vi "DefaultFromINI.vi"(8 "error in (no error)":errorcluster, 11 "ChromaPowerSupply":refnum<class "ChromaPowerSupply.lvclass">) -> (0 "error out":errorcluster, 3 "ChromaPowerSupply":refnum<class "ChromaPowerSupply.lvclass">)   [LabVIEW 2018, in "AcPwrPlugins.lvlib" / "ChromaPowerSupply.lvclass"]
doc: "This VI loads the instruments' configuration previously stored on file."
uses:
  ChromaPowerSupply.lvclass
  C:/Program Files (x86)/National Instruments/LabVIEW 2018/user.lib/NIST/BaseClasses/BasePlugin_class/BasePlugin.lvclass
  C:/Users/Public/Projects/ICDAS/NistPluggableModules/AcPwr/AcPwrPlugins/AcPwrBaseClass/AcPwrBase.lvclass
  TypeDefs/Device(s)Settings.ctl
  TypeDefs/Measurements.ctl
  <userlib>/NIST/BaseClasses/BasePlugin_class/BasePlugin.lvclass/BasePlugin.ctl
  <userlib>/NIST/BaseClasses/BasePlugin_class/Accessors/Read PluginIniFilePath.vi
  AcPwrBaseClass/AcPwrBase.lvclass
  <vilib>/Utility/config.llb/NI_LVConfig.lvlib
  TestClass/Test.lvclass
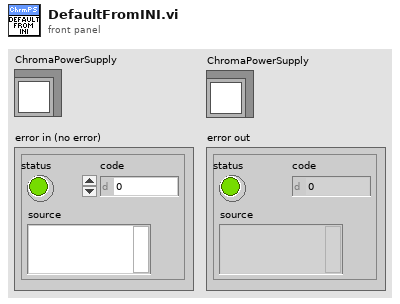
[diagram p1: front panel]
types:
  T1 = typedef "AcPwrPlugins.lvlib/ChromaPowerSupply.lvclass/Measurements.ctl" = cluster{"Handle":string, "Name":string, "Enabled":bool, "Measurement Value":dbl, "btnMeasFetch":bool, "ProtectionStatusString":string, "Measurement Type":i32}[]
  T2 = typedef "AcPwrPlugins.lvlib/ChromaPowerSupply.lvclass/Device(s)Settings.ctl" = cluster{"Phases":cluster{"Handle":string, "Instrument Options":string, "id query (T)":bool, "reset device (T)":bool, "Timing":cluster{"TimingOn":enum16{""}, "Hours":u32, "Minutes":u32, "Seconds":dbl, "CutoffVoltage":dbl}, "Connected":bool, "Output Mode":enum16{"Voltage (DC)", "Current (DC)"}, "Voltage":dbl, "Current":dbl, "Voltage Limit":dbl, "Current Limit":dbl, "Power Protect":dbl, "Current Protect":dbl, "Voltage Protect":dbl}[], "MeasName":string}
  T3 = typedef "NI_LVConfig.lvlib/Config Data RefNum.ctl" = refnum<k1>
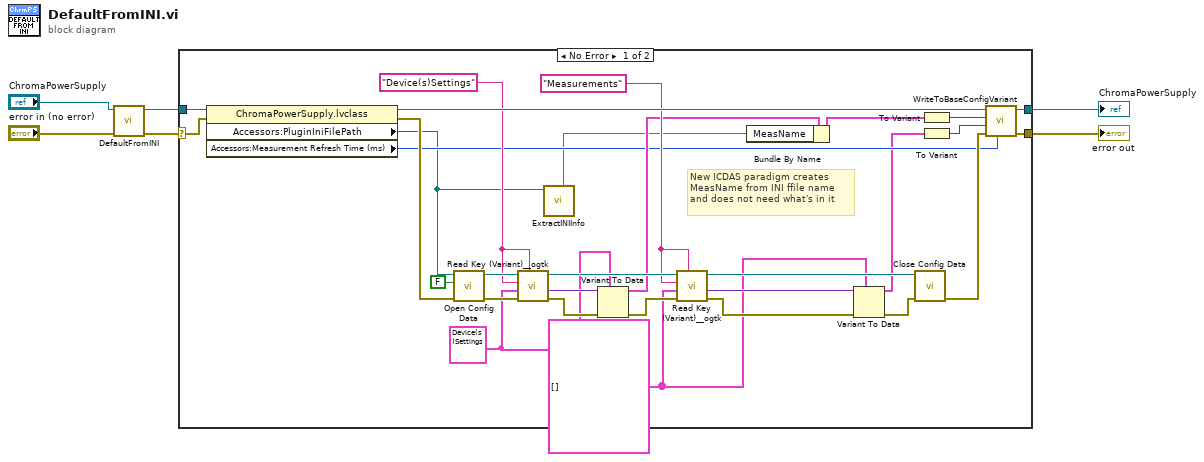
[diagram p0: block diagram]
diagram:
  n1 = call-parent "DefaultFromINI.vi"("error in (no error)"="error in (no error)", "AcPwrBase"="ChromaPowerSupply") -> ("error out"=w4:errorcluster, "AcPwrBase"=w3:refnum<class "ChromaPowerSupply.lvclass">)  [unwired: 8 in]
  n2 = case shown="No Error" w4 {
    selector: w4 -> [w28 w37]
    tunnel: w3 -> [w36 w38]
    tunnel: [w17 w38] -> w2
    tunnel: [w16 w37] -> w1
    frame No Error {
      w11 = T1 [] ("Measurements")
      w12 = T2 {"Phases"=[{"Handle"="", "Instrument Options"="", "id query (T)"=TRUE, "reset device (T)"=TRUE, "Timing"={"TimingOn"=enum."", "Hours"=0, "Minutes"=0, "Seconds"=0.0, "CutoffVoltage"=0.0}, "Connected"=FALSE, "Output Mode"=enum."Voltage (DC)", "Voltage"=0.0, "Current"=0.0, "Voltage Limit"=0.0, "Current Limit"=0.0, "Power Protect"=0.0, "Current Protect"=0.0, "Voltage Protect"=0.0}], "MeasName"=""} ("Device(s)Settings")
      w19 = "Measurements" ("section")
      w29 = "Device(s)Settings" ("section")
      # "New ICDAS paradigm creates\nMeasName from INI ffile name\nand does not need what's in it"
      n3 = property class="ChromaPowerSupply.lvclass"(reference=w36, error in=w28) -> (reference out=w30:refnum<class "ChromaPowerSupply.lvclass">, error out=w27:errorcluster, "Accessors:PluginIniFilePath"=w10:path, "Accessors:Measurement Refresh Time (ms)"=w14:u32)
      n4 = call <vilib>:"Open Config Data.vi"("error in (no error)"=w27, "create file if necessary (T)"=FALSE, "configuration file path"=w10) -> ("error out"=w33:errorcluster, "refnum"=w34:T3)  [unwired: 6 in, 1 out]
      n5 = call <userlib>:"Read Key (Variant)__ogtk.vi"("section"=w29, "error in (no error)"=w33, "type"=w12, "key (optional)"=w29, "refnum"=w34) -> ("error out"=w31:errorcluster, "key-value"=w32:variant, "refnum out"=w23:T3)  [unwired: 3 in, 1 out]
      n6 = call "ExtractINIInfo.vi"("INI File Path"=w10) -> ("Module.Class.INI File Name"=w7:string)  [unwired: 4 in, 6 out]
      n7 = Variant To Data(error in=w31, type=w12, Variant=w32) -> (data=w15:T2, error out=w20:errorcluster)
      n8 = call <userlib>:"Read Key (Variant)__ogtk.vi"("section"=w19, "error in (no error)"=w20, "type"=w11, "key (optional)"=w19, "refnum"=w23) -> ("error out"=w25:errorcluster, "key-value"=w24:variant, "refnum out"=w22:T3)  [unwired: 3 in, 1 out]
      n9 = Bundle By Name(cluster=w15, "MeasName"=w7) -> (w8:T2)
      n10 = Variant To Data(error in=w25, type=w11, Variant=w24) -> (data=w9:T1, error out=w21:errorcluster)
      n11 = call <vilib>:"Close Config Data.vi"("error in (no error)"=w21, "refnum"=w22) -> ("error out"=w26:errorcluster)  [unwired: 8 in, 1 out]
      n12 = To Variant(anything=w8) -> (Variant=w18:variant)
      n13 = To Variant(anything=w9) -> (Variant=w13:variant)
      n14 = call-dynamic "WriteToBaseConfigVariant.vi"("Measurement Refresh Time (ms)"=w14, "error in (no error)"=w26, "Meas"=w13, "Config"=w18, "ChromaPowerSupply in"=w30) -> ("error out"=w16:errorcluster, "ChromaPowerSupply out"=w17:refnum<class "ChromaPowerSupply.lvclass">)  [unwired: 5 in]
    }
    frame Error {
    }
  }
  "error out" <- w1
  "ChromaPowerSupply" <- w2
